vi "Main.vi"() -> ()   [LabVIEW 2020]
doc: "QMH calculatrice"
uses:
  controls/UI Data.ctl
  support/Message Queue/Enqueue Message (Single).vi
  <vilib>/Utility/error.llb/Error Cluster From Error Code.vi
  <vilib>/ErrorRing/Error Ring.xnode
  support/Message Queue/Message Queue.lvlib
  support/User Event - Stop/User Event - Stop.lvlib
panel:
  in  "Btn_Error_2":bool caption="Error state"
  in  "Btn_Error_1":bool caption="Error 1"
  out "sortie d'erreur":errorcluster
  out "Display":cluster{"Num":dbl, "Char":string}
  in  "Pad":T1
  in  "Btn_Stop":bool
  # "Calculatrice"
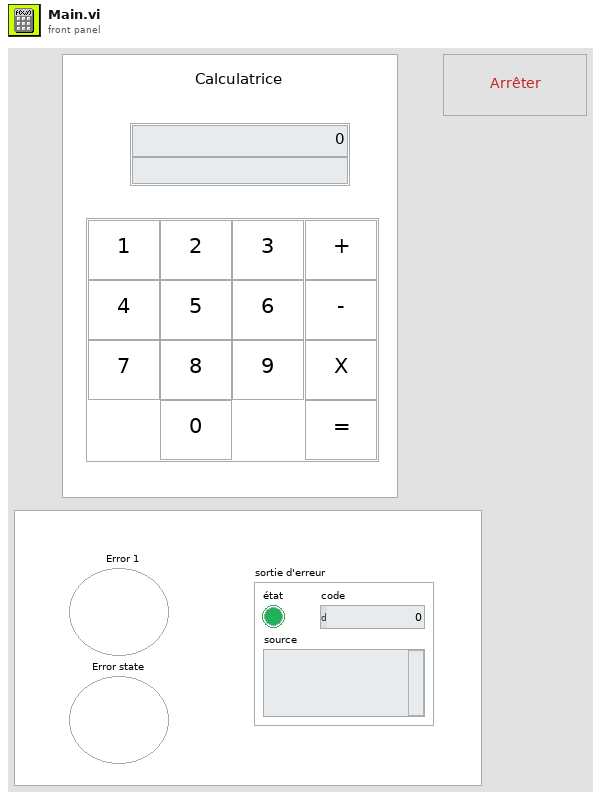
[diagram p1: front panel]
types:
  T1 = cluster{"Btn_1":bool, "Btn_2":bool, "Btn_3":bool, "Btn_4":bool, "Btn_5":bool, "Btn_6":bool, "Btn_7":bool, "Btn_8":bool, "Btn_9":bool, "Btn_0":bool, "Btn_+":bool, "Btn_-":bool, "Btn_X":bool, "Btn_=":bool}
  T2 = cluster{"état":bool, "code":i32, "source":string}
  T3 = typedef "Message Queue.lvlib/All Message Queues.ctl" = cluster{"IU":refnum<queue>}
  T4 = typedef "UI Data.ctl" = cluster{"Char_mem":string, "Réf du bouton Quitter":refnum<vi>, "Display":cluster{"Num":dbl, "Char":string}, "Event":cluster{"Stop":refnum<user-event>}}
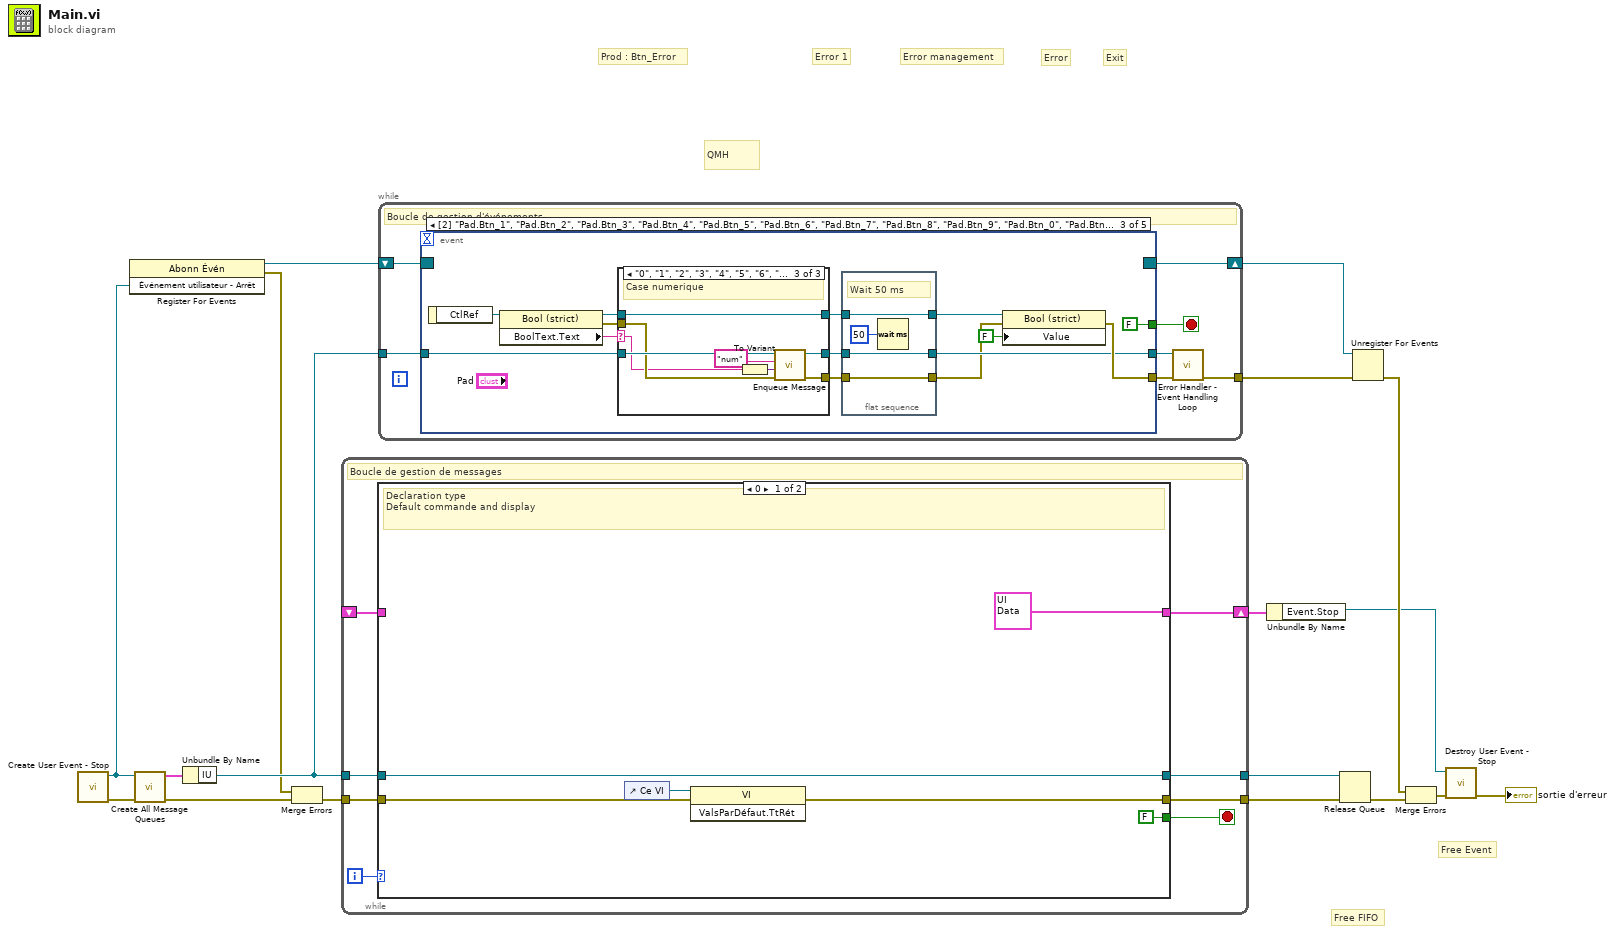
[diagram p0: block diagram]
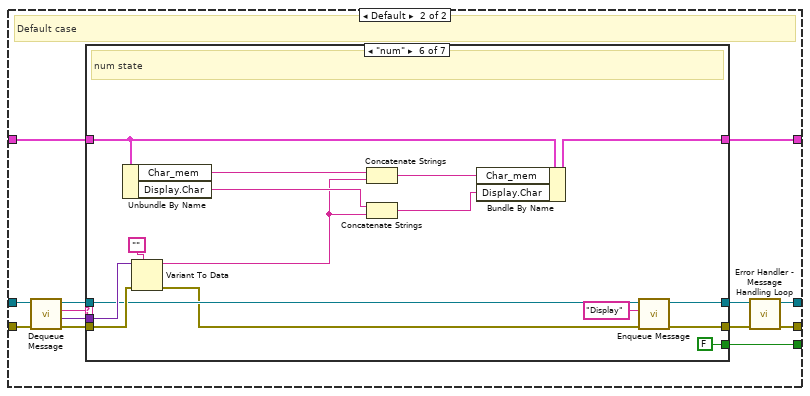
[diagram p2: hidden frame]
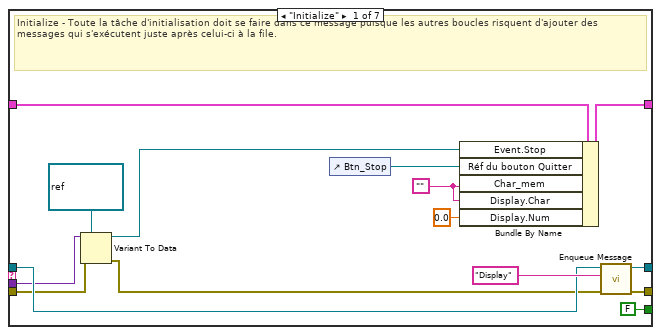
[diagram p3: hidden frame]
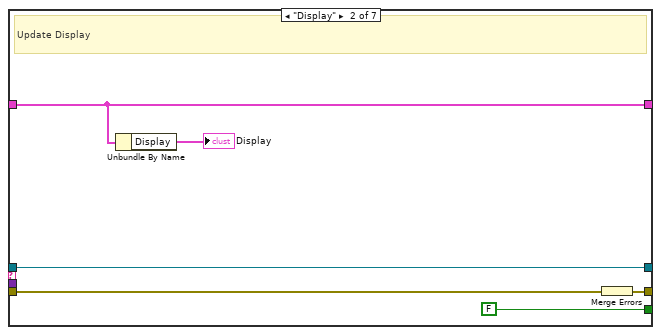
[diagram p4: hidden frame]
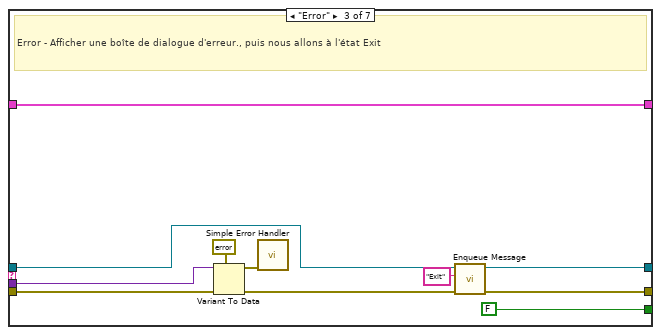
[diagram p5: hidden frame]
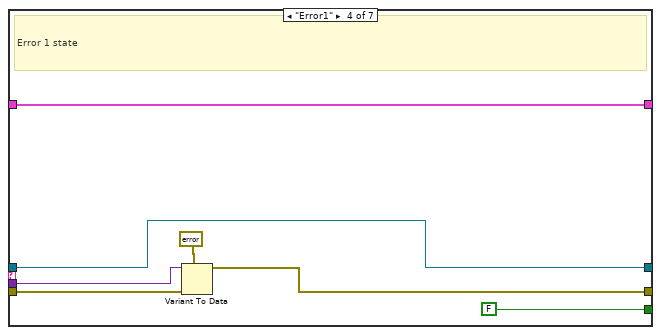
[diagram p6: hidden frame]
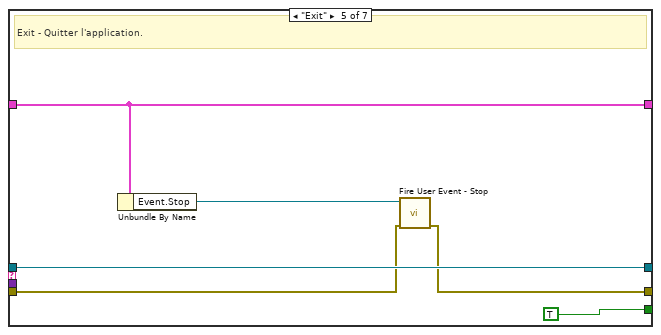
[diagram p7: hidden frame]
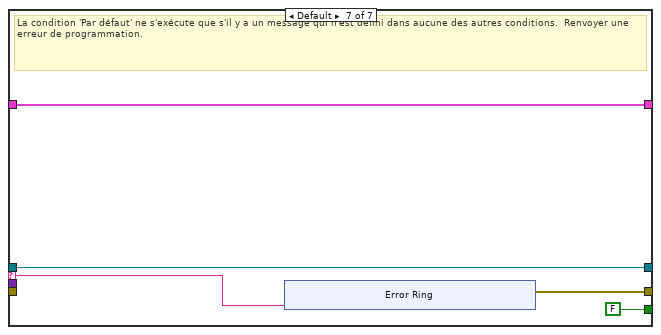
[diagram p8: hidden frame]
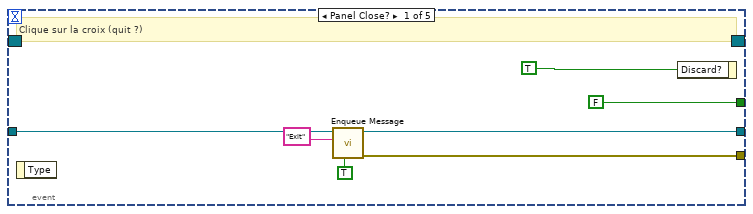
[diagram p9: hidden frame]
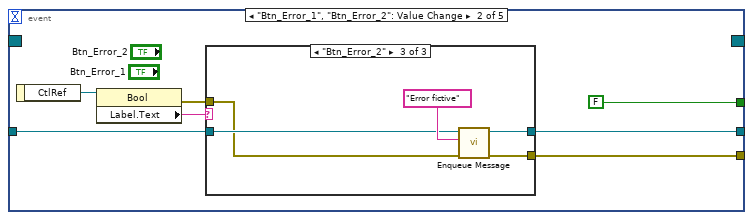
[diagram p10: hidden frame]
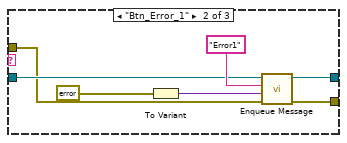
[diagram p12: hidden frame]
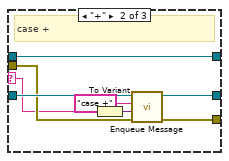
[diagram p14: hidden frame]
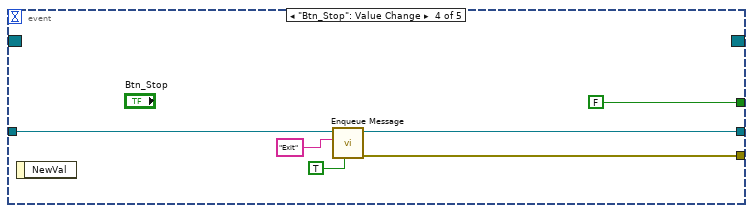
[diagram p15: hidden frame]
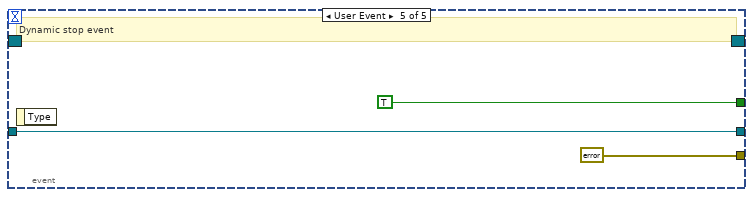
[diagram p16: hidden frame]
diagram:
  # "Free Event"
  # "Free FIFO"
  # "Exit"
  # "Error"
  # "Error management"
  # "Prod : Btn_Error"
  # "Error 1"
  # "QMH"
  n1 = call "Create User Event - Stop.vi"() -> ("error out"=w15:T2, "Événement utilisateur - Arrêt"=w3:refnum<user-event>)  [unwired: 10 in]
  n2 = register-events(w3) -> (reference out=w10:refnum<event-registration>, error out=w8:errorcluster)  [unwired: 2 in]
  n3 = call "Create All Message Queues.vi"("error in (no error)"=w15, "Événement utilisateur - Arrêt"=w3) -> ("error out"=w18:T2, "Files d'attente de messages en sortie"=w17:T3)  [unwired: 8 in]
  n4 = Unbundle By Name(w17) -> ("IU"=w16:refnum<queue>)
  n5 = Merge Errors(w8, w18) -> (w9:errorcluster)
  n6 = while {
    tunnel: w16 -> [w22]
    shift-right: [w25] -> w2
    shift-left: _ -> [w26]
    tunnel: w9 -> [w23]
    tunnel: [w21] -> w6
    tunnel: [w20] -> w4
    i -> [w19]
    stop <- w24 stop-if-true
    # "Boucle de gestion de messages"
    n7 = case shown="0" w19 {
      tunnel: w26 -> [_ w45]
      tunnel: [T4 {"Char_mem"="", "Réf du bouton Quitter"=refnum, "Display"={"Num"=0.0, "Char"=""}, "Event"={"Stop"=refnum}} ("Data Cluster") w44] -> w25
      tunnel: [FALSE w43] -> w24
      tunnel: w23 -> [w28 w42]
      tunnel: w22 -> [w31 w38]
      tunnel: [w27 w36] -> w21
      tunnel: [w31 w33] -> w20
      frame 0 {
        # "Declaration type\nDefault commande and display"
        n8 = control-ref of="Ce VI"() -> (w29:refnum<vi>)
        n9 = invoke class="VI" method="ValsParDéfaut.TtRét"(reference=w29, error in=w28) -> (error out=w27:errorcluster)  [unwired: 1 in, 2 out]
      }
      frame Default {
        # "Default case"
        n10 = call "Dequeue Message.vi"("error in (no error)"=w42, "File d'attente de messages"=w38) -> ("error out"=w41:T2, "Données de message"=w39:variant, "Message"=w40:string, "File d'attente de message dup."=w37:refnum<queue>)  [unwired: 6 in]
        n11 = case "Conditions des messages" shown="\"num\"" w40 {
          selector: w40 -> [_ _ _ _ _ _ w109]
          tunnel: w37 -> [w55 w65 w68 w78 w89 w96 w108]
          tunnel: w41 -> [w51 w63 w77 w84 w88 w104 _]
          tunnel: [w60 w66 w69 w80 w87 w94 w110] -> w35
          tunnel: w45 -> [w59 w62 w76 w83 w86 w103 w111]
          tunnel: [w58 w62 w76 w83 w86 w99 w111] -> w44
          tunnel: [FALSE FALSE FALSE FALSE TRUE FALSE FALSE] -> w43
          tunnel: w39 -> [w52 _ w75 w82 _ w106 _]
          tunnel: [w54 w65 w67 w78 w89 w95 w108] -> w34
          frame "Initialize" {
            w47 = ""
            # "Initialize - Toute la tâche d'initialisation doit se faire dans ce message puisque les autres boucles risquent d'ajouter des messages qui s'exécutent juste après celui-ci à la file."
            n12 = Variant To Data(error in=w51, type=refnum<user-event> refnum ("Événement utilisateur - Arrêt"), Variant=w52) -> (data=w49:refnum<user-event>, error out=w48:errorcluster)
            n13 = control-ref of="Btn_Stop"() -> (w57:refnum<vi>)
            n14 = Bundle By Name(cluster=w59, "Event.Stop"=w49, "Réf du bouton Quitter"=w57, "Char_mem"=w47, "Display.Char"=w47, "Display.Num"=0.0) -> (w58:T4)
            n15 = call-poly "Enqueue Message.vi"("error in (no error)"=w48, "Message"="Display", "File d'attente de messages"=w55) -> ("error out"=w60:T2, "File d'attente de message dup."=w54:refnum<queue>)  [unwired: 7 in]
          }
          frame "Display" {
            # "Update Display"
            n16 = Unbundle By Name(w62) -> ("Display"=→"Display":cluster{"Num":dbl, "Char":string})
            n17 = Merge Errors(w63) -> (w66:errorcluster)
          }
          frame "Error" {
            # "Error - Afficher une boîte de dialogue d'erreur., puis nous allons à l'état Exit"
            n18 = Variant To Data(error in=w77, type=errorcluster {"status"=FALSE, "code"=0, "source"=""} ("error constant"), Variant=w75) -> (data=w73:errorcluster, error out=w70:errorcluster)
            n19 = call <vilib>:"Simple Error Handler.vi"("error in (no error)"=w73) -> ()  [unwired: 4 in, 5 out]
            n20 = call-poly "Enqueue Message.vi"("error in (no error)"=w70, "Message"="Exit", "File d'attente de messages"=w68) -> ("error out"=w69:T2, "File d'attente de message dup."=w67:refnum<queue>)  [unwired: 7 in]
          }
          frame "Error1" {
            # "Error 1 state"
            n21 = Variant To Data(error in=w84, type=errorcluster {"status"=FALSE, "code"=0, "source"=""} ("error constant"), Variant=w82) -> (data=w80:errorcluster)  [unwired: 1 out]
          }
          frame "Exit" {
            # "Exit - Quitter l'application."
            n22 = Unbundle By Name(w86) -> ("Event.Stop"=w85:refnum<user-event>)
            n23 = call "Fire User Event - Stop.vi"("error in (no error)"=w88, "Événement utilisateur - Arrêt"=w85) -> ("error out"=w87:T2)  [unwired: 9 in]
          }
          frame "num" {
            # "num state"
            n24 = Unbundle By Name(w103) -> ("Char_mem"=w102:string, "Display.Char"=w101:string)
            n25 = Variant To Data(error in=w104, type="", Variant=w106) -> (data=w100:string, error out=w92:errorcluster)
            n26 = Concatenate Strings(w102, w100) -> (w98:string)
            n27 = Concatenate Strings(w101, w100) -> (w97:string)
            n28 = Bundle By Name(cluster=w103, "Char_mem"=w98, "Display.Char"=w97) -> (w99:T4)
            n29 = call-poly "Enqueue Message.vi"("error in (no error)"=w92, "Message"="Display", "File d'attente de messages"=w96) -> ("error out"=w94:T2, "File d'attente de message dup."=w95:refnum<queue>)  [unwired: 7 in]
          }
          frame Default {
            # "La condition 'Par défaut' ne s'exécute que s'il y a un message qui n'est défini dans aucune des autres conditions.  Renvoyer une erreur de programmation."
            n30 = xnode ("Error Ring")("paramètre 0"=w109) -> ("sortie d'erreur"=w110:errorcluster)
          }
        }
        n31 = call "Error Handler - Message Handling Loop.vi"("error in (no error)"=w35, "File d'attente de messages"=w34) -> ("erreur en entrée dup."=w36:T2, "File d'attente de message dup."=w33:refnum<queue>)  [unwired: 8 in]
      }
    }
  }
  n32 = while {
    tunnel: w16 -> [w125]
    shift-right: [w123] -> w12
    shift-left: w10 -> [w124]
    tunnel: [w119] -> w11
    stop <- w121 stop-if-true
    # "Boucle de gestion d'événements"
    n33 = event shown="[2] \"Pad.Btn_1\", \"Pad.Btn_2\", \"Pad.Btn_3\", \"Pad.Btn_4\", \"Pad.Btn_5\", \"Pad.Btn_6\", \"Pad.Btn_7\", \"Pad.Btn_8\", \"Pad.Btn_9\", \"Pad.Btn_0\", \"Pad.Btn_+\": Valeur changée" {
      selector: w124 -> [_ _ _ _ _]
      dyn-events: [_ _ _ _ _] -> w123
      timeout: _ -> [_ _ _ _ _]
      tunnel: [FALSE ("Discard?") FALSE ("Discard?") FALSE ("Discard?") FALSE ("Discard?") TRUE ("Discard?")] -> w121
      tunnel: w125 -> [w131 w139 w167 w196 w199]
      tunnel: [w130 w137 w162 w195 T2 {"état"=FALSE, "code"=0, "source"=""} ("error out")] -> w122
      tunnel: [w129 w138 w155 w194 w199] -> w120
      event Panel Close? {
        # "Clique sur la croix (quit ?)"
        n34 = event-data() -> ()  [unwired: 1 in, 1 out]
        n35 = call-poly "Enqueue Message.vi"("Message prioritaire ? (F)"=TRUE ("Priority Message? (F)"), "Message"="Exit", "File d'attente de messages"=w131) -> ("error out"=w130:T2, "File d'attente de message dup."=w129:refnum<queue>)  [unwired: 7 in]
        n36 = event-data ("Event Filter Node")("Discard?"=TRUE) -> ()  [unwired: 1 in, 1 out]
      }
      event "Btn_Error_1", "Btn_Error_2": Value Change {
        n37 = event-data() -> ("CtlRef"=w135:refnum<vi>)  [unwired: 1 in]
        n38 = property class="Bool"(reference=w135) -> (error out=w133:errorcluster, "Label.Text"=w134:string)  [unwired: 1 in, 1 out]
        n39 = case shown="\"Btn_Error_2\"" w134 {
          tunnel: w139 -> [w141 w147 w152]
          tunnel: [w141 w146 w151] -> w138
          tunnel: [w140 w145 w150] -> w137
          tunnel: w133 -> [w140 w142 w149]
          frame Default {
          }
          frame "Btn_Error_1" {
            n40 = To Variant(anything=T2 {"état"=TRUE, "code"=500, "source"="Voici error 1"} ("error out")) -> (Variant=w143:variant)
            n41 = call-poly "Enqueue Message.vi"("error in (no error)"=w142, "Données de message"=w143, "Message"="Error1", "File d'attente de messages"=w147) -> ("error out"=w145:T2, "File d'attente de message dup."=w146:refnum<queue>)  [unwired: 6 in]
          }
          frame "Btn_Error_2" {
            n42 = call-poly "Enqueue Message.vi"("error in (no error)"=w149, "Message"="Error fictive", "File d'attente de messages"=w152) -> ("error out"=w150:T2, "File d'attente de message dup."=w151:refnum<queue>)  [unwired: 7 in]
          }
        }
      }
      event "Pad.Btn_1", "Pad.Btn_2", "Pad.Btn_3", "Pad.Btn_4", "Pad.Btn_5", "Pad.Btn_6", "Pad.Btn_7", "Pad.Btn_8", "Pad.Btn_9", "Pad.Btn_0", "Pad.Btn_+": Value Change {
        n43 = event-data() -> ("CtlRef"=w165:refnum<vi>)  [unwired: 1 in]
        n44 = property class="Bool (strict)"(reference=w165) -> (reference out=w161:refnum<vi>, error out=w163:errorcluster, "BoolText.Text"=w164:string)  [unwired: 1 in]
        n45 = case shown="\"0\", \"1\", \"2\", \"3\", \"4\", \"5\", \"6\", \"7\", \"8\", \"9\"" w164 {
          selector: w164 -> [_ w177 w185]
          tunnel: w167 -> [w174 w181 w189]
          tunnel: [w174 w180 w188] -> w158
          tunnel: [w173 w179 w187] -> w159
          tunnel: w163 -> [w173 w178 w186]
          tunnel: w161 -> [w172 w175 w183]
          tunnel: [w172 w175 w183] -> w157
          frame Default {
          }
          frame "+" {
            # "case +"
            n46 = To Variant(anything=w177) -> (Variant=w176:variant)
            n47 = call-poly "Enqueue Message.vi"("error in (no error)"=w178, "Données de message"=w176, "Message"="case +", "File d'attente de messages"=w181) -> ("error out"=w179:T2, "File d'attente de message dup."=w180:refnum<queue>)  [unwired: 6 in]
          }
          frame "0", "1", "2", "3", "4", "5", "6", "7", "8", "9" {
            # "Case numerique"
            n48 = To Variant(anything=w185) -> (Variant=w184:variant)
            n49 = call-poly "Enqueue Message.vi"("error in (no error)"=w186, "Données de message"=w184, "Message"="num", "File d'attente de messages"=w189) -> ("error out"=w187:T2, "File d'attente de message dup."=w188:refnum<queue>)  [unwired: 6 in]
          }
        }
        n50 = flat-sequence {
          tunnel: w159 -> [w169]
          tunnel: w158 -> [w170]
          tunnel: w157 -> [w171]
          tunnel: [w171] -> w156
          tunnel: [w170] -> w155
          tunnel: [w169] -> w154
          frame #0 {
            # "Wait 50 ms"
            n51 = Wait (ms)(milliseconds to wait=u32 50 ("attente (ms)")) -> ()  [unwired: 1 out]
          }
        }
        n52 = property class="Bool (strict)"(reference=w156, error in=w154, "Value"=FALSE ("Valeur")) -> (error out=w162:errorcluster)  [unwired: 1 out]
      }
      event "Btn_Stop": Value Change {
        n53 = event-data() -> ()  [unwired: 1 in, 1 out]
        n54 = call-poly "Enqueue Message.vi"("Message prioritaire ? (F)"=TRUE ("Priority Message? (F)"), "Message"="Exit", "File d'attente de messages"=w196) -> ("error out"=w195:T2, "File d'attente de message dup."=w194:refnum<queue>)  [unwired: 7 in]
      }
      event User Event {
        # "Dynamic stop event"
        n55 = event-data() -> ()  [unwired: 1 in, 1 out]
      }
    }
    n56 = call "Error Handler - Event Handling Loop.vi"("error in (no error)"=w122, "File d'attente de messages"=w120) -> ("erreur en entrée dup."=w119:T2)  [unwired: 8 in, 1 out]
  }
  n57 = Unbundle By Name(w2) -> ("Event.Stop"=w1:refnum<user-event>)
  n58 = Release Queue(queue=w4, error in (no error)=w6) -> (error out=w5:errorcluster)  [unwired: 1 in, 2 out]
  n59 = Unregister For Events(event registration refnum=w12, error in=w11) -> (error out=w13:errorcluster)
  n60 = Merge Errors(w13, w5) -> (w14:errorcluster)
  n61 = call "Destroy User Event - Stop.vi"("error in (no error)"=w14, "Événement utilisateur - Arrêt"=w1) -> ("error out"=→"sortie d'erreur":T2)  [unwired: 9 in]
